vi "ComputeTargeting.vi"(6 "Reset PID":bool, 7 "Target Mid (Default High)":bool, 8 "error in (no error)":errorcluster, 11 "Sorted Target Info":T4) -> (0 "error out":errorcluster, 1 "Flattened Data":string, 2 "Y Axis Value":dbl, 3 "X Axis Value":dbl)   [LabVIEW 2011]
uses:
  <vilib>/addons/control/pid/pid.llb/PID (DBL).vi
  <vilib>/addons/control/pid/NI_PID_pid.lvlib
panel:
  in  "Cluster":T1
  out "Chosen Target":T2
  in  "PID gains":T3={"proportional gain (Kc)"=1.0, "integral time (Ti, min)"=0.01, "derivative time (Td, min)"=0.0} {"derivative time (Td, min)" format="%.3f"; "integral time (Ti, min)" format="%.3f"; "proportional gain (Kc)" format="%.3f"}
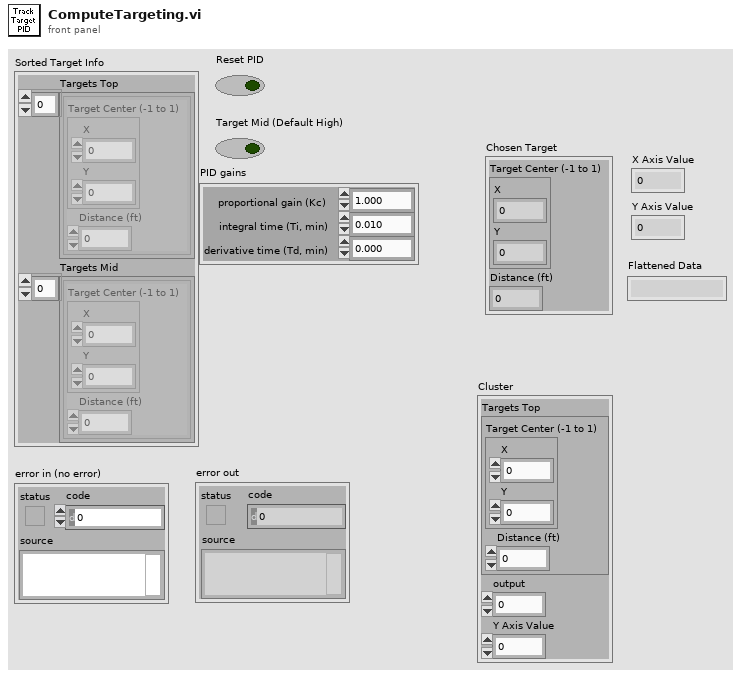
[diagram p1: front panel]
types:
  T1 = cluster{"Targets Top":cluster{"Target Center (-1 to 1)":cluster{"X":dbl, "Y":dbl}, "Distance (ft)":dbl}, "output":dbl, "Y Axis Value":dbl}
  T2 = cluster{"Target Center (-1 to 1)":cluster{"X":dbl, "Y":dbl}, "Distance (ft)":dbl}
  T3 = cluster{"proportional gain (Kc)":dbl, "integral time (Ti, min)":dbl, "derivative time (Td, min)":dbl}
  T4 = cluster{"Targets Top":cluster{"Target Center (-1 to 1)":cluster{"X":dbl, "Y":dbl}, "Distance (ft)":dbl}[], "Targets Mid":cluster{"Target Center (-1 to 1)":cluster{"X":dbl, "Y":dbl}, "Distance (ft)":dbl}[]}
  T5 = cluster{"Target Center (-1 to 1)":cluster{"X":dbl, "Y":dbl}, "Distance (ft)":dbl}[]
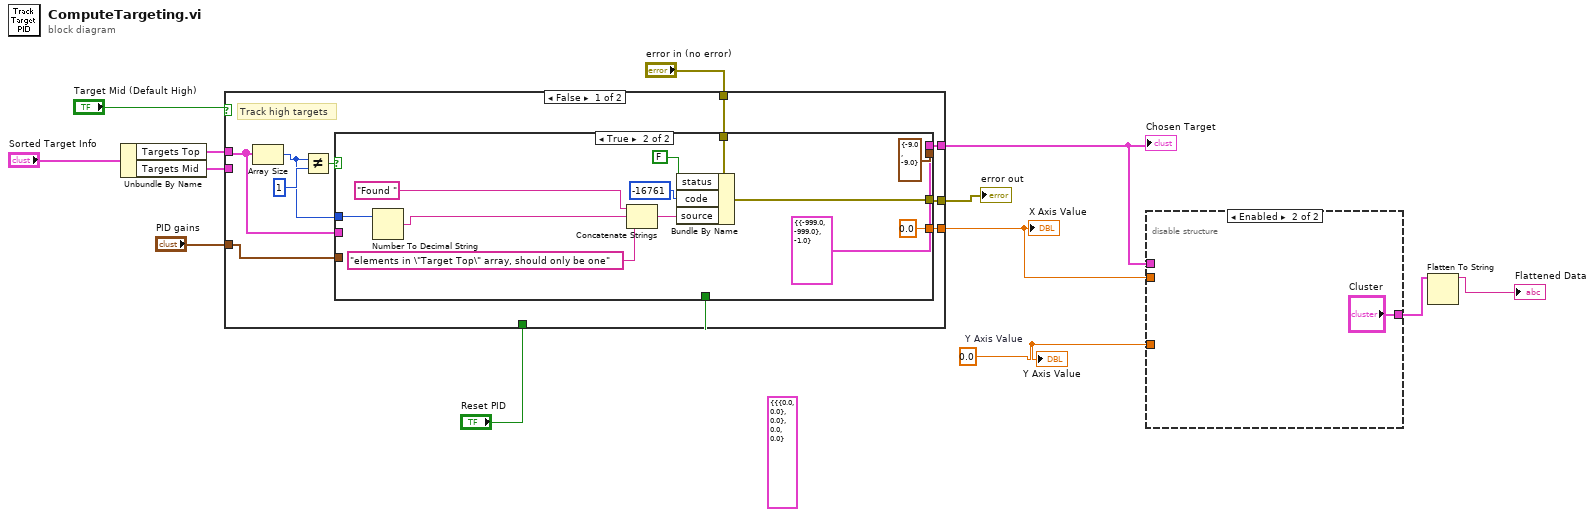
[diagram p0: block diagram]
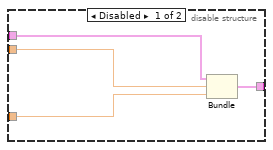
[diagram p2: hidden frame]
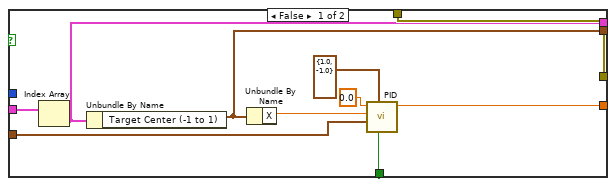
[diagram p3: hidden frame]
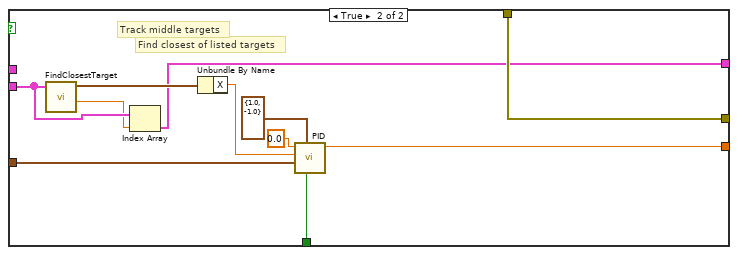
[diagram p4: hidden frame]
diagram:
  (unwired) T1 {"Targets Top"={"Target Center (-1 to 1)"={"X"=0.0, "Y"=0.0}, "Distance (ft)"=0.0}, "output"=0.0, "Y Axis Value"=0.0} ("output cluster")
  w3 = 0.0  # Y Axis Value
  n1 = Unbundle By Name("Sorted Target Info") -> ("Targets Top"=w11:T5, "Targets Mid"=w10:T5)
  n2 = case shown="False" "Target Mid (Default High)" {
    tunnel: w11 -> [w18 _]
    tunnel: w10 -> [_ w48]
    tunnel: "error in (no error)" -> [w21 w49]
    tunnel: "PID gains" -> [w15 w55]
    tunnel: "Reset PID" -> [w16 w54]
    tunnel: [w17 w52] -> w2
    tunnel: [w19 w49] -> w6
    tunnel: [w14 w46] -> w4
    frame False {
      # "Track high targets"
      n3 = Array Size(array=w18) -> (size(s)=w20:i32)
      n4 = Not Equal?(x=w20, y=1) -> (x != y?=w22:bool)
      n5 = case shown="True" w22 {
        tunnel: w21 -> [w33 w45]
        tunnel: w20 -> [_ w44]
        tunnel: [w33 w37] -> w19
        tunnel: w18 -> [w30 _]
        tunnel: [w29 0.0 ("output")] -> w17
        tunnel: w16 -> [w28 _]
        tunnel: w15 -> [w27 _]
        tunnel: [w26 cluster{"X":dbl, "Y":dbl} {"X"=-9.0, "Y"=-9.0} ("Target Center (-1 to 1)")] -> _
        tunnel: [w24 T2 {"Target Center (-1 to 1)"={"X"=-999.0, "Y"=-999.0}, "Distance (ft)"=-1.0} ("Targets Top")] -> w14
        frame False {
          n6 = Index Array(array=w30) -> (element=w24:T2)  [unwired: 1 in]
          n7 = Unbundle By Name(w24) -> ("Target Center (-1 to 1)"=w26:cluster{"X":dbl, "Y":dbl})
          n8 = Unbundle By Name(w26) -> ("X"=w25:dbl)
          n9 = call-poly <vilib>:"PID.vi"("reinitialize? (F)"=w28, "output range"=cluster{"output high":dbl, "output low":dbl} {"output high"=1.0, "output low"=-1.0}, "PID gains"=w27, "process variable"=w25, "setpoint"=0.0) -> ("output"=w29:dbl)  [unwired: 5 in, 1 out]
        }
        frame True {
          n10 = Number To Decimal String(number=w44) -> (decimal integer string=w42:string)  [unwired: 1 in]
          n11 = Concatenate Strings("Found ", w42, "elements in \"Target Top\" array, should only be one") -> (w40:string)
          n12 = Bundle By Name(cluster=w45, "status"=FALSE, "code"=-16761, "source"=w40) -> (w37:errorcluster)
        }
      }
    }
    frame True {
      # "Find closest of listed targets"
      # "Track middle targets"
      n13 = call "FindClosestTarget.vi"("Targets To Sort"=w48) -> ("Index"=w47:dbl, "Target Center (-1 to 1)"=w50:cluster{"X":dbl, "Y":dbl})  [unwired: 8 in, 1 out]
      n14 = Index Array(array=w48, index=w47) -> (element=w46:T2)
      n15 = Unbundle By Name(w50) -> ("X"=w53:dbl)
      n16 = call-poly <vilib>:"PID.vi"("reinitialize? (F)"=w54, "output range"=cluster{"output high":dbl, "output low":dbl} {"output high"=1.0, "output low"=-1.0}, "PID gains"=w55, "process variable"=w53, "setpoint"=0.0) -> ("output"=w52:dbl)  [unwired: 5 in, 1 out]
    }
  }
  "X Axis Value" <- w2
  "error out" <- w6
  "Chosen Target" <- w4
  n17 = disable-structure shown="Enabled" {
    disable-tunnel: w4 -> [w60 _]
    disable-tunnel: w3 -> [w58 _]
    disable-tunnel: w2 -> [w59 _]
    disable-tunnel: [w57 "Cluster"] -> w1
    frame Disabled {
      n18 = Bundle("Targets Top"=w60, "output"=w59, "Y Axis Value"=w58) -> (w57:T1)  [unwired: 1 in]
    }
    frame Enabled {
    }
  }
  n19 = Flatten To String(anything=w1) -> (data string=→"Flattened Data":string)  [unwired: 3 in, 2 out]
  "Y Axis Value" <- w3
